vi "getThermocouplesamples.vi"(8 "error in":errorcluster, 11 "params":refnum<class "JSON Value.lvclass">) -> (0 "error out":errorcluster, 3 "data":refnum<class "JSON Value.lvclass">)   [LabVIEW 2017]
uses:
  <vilib>/NI/JSON Support for LabVIEW/JSON Value/JSON Value.lvclass
  <vilib>/DAQmx/read.llb/DAQmx Read (Analog 1D DBL 1Chan NSamp).vi
  <vilib>/NI/JSON Support for LabVIEW/JSON Value/Object/Get Value/Get Value (String).vi
  <vilib>/NI/JSON Support for LabVIEW/JSON Value/Object/Get Value/Get Value (Numeric).vi
  <vilib>/DAQmx/create/channels.llb/DAQmx Create Channel (AI-Temperature-Thermocouple).vi
  <vilib>/DAQmx/configure/timing.llb/DAQmx Timing (Sample Clock).vi
  <vilib>/DAQmx/miscellaneous.llb/DAQmx Fill In Error Info.vi
  <vilib>/NI/JSON Support for LabVIEW/JSON Value/New JSON Value/New JSON (Numeric[]).vi
  <vilib>/NI/JSON Support for LabVIEW/JSON Value/New JSON Value/New JSON (Numeric).vi
  <vilib>/NI/JSON Support for LabVIEW/JSON Value/New JSON Value/New JSON ({Value[]}).vi
  <vilib>/NI/NI JSONRPC Server Framework/Classes/Server/JSONRPC Server.lvclass
  <resource>/objmgr/daqmx.rc
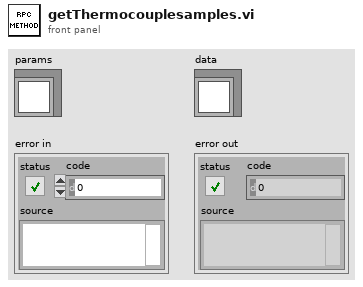
[diagram p1: front panel]
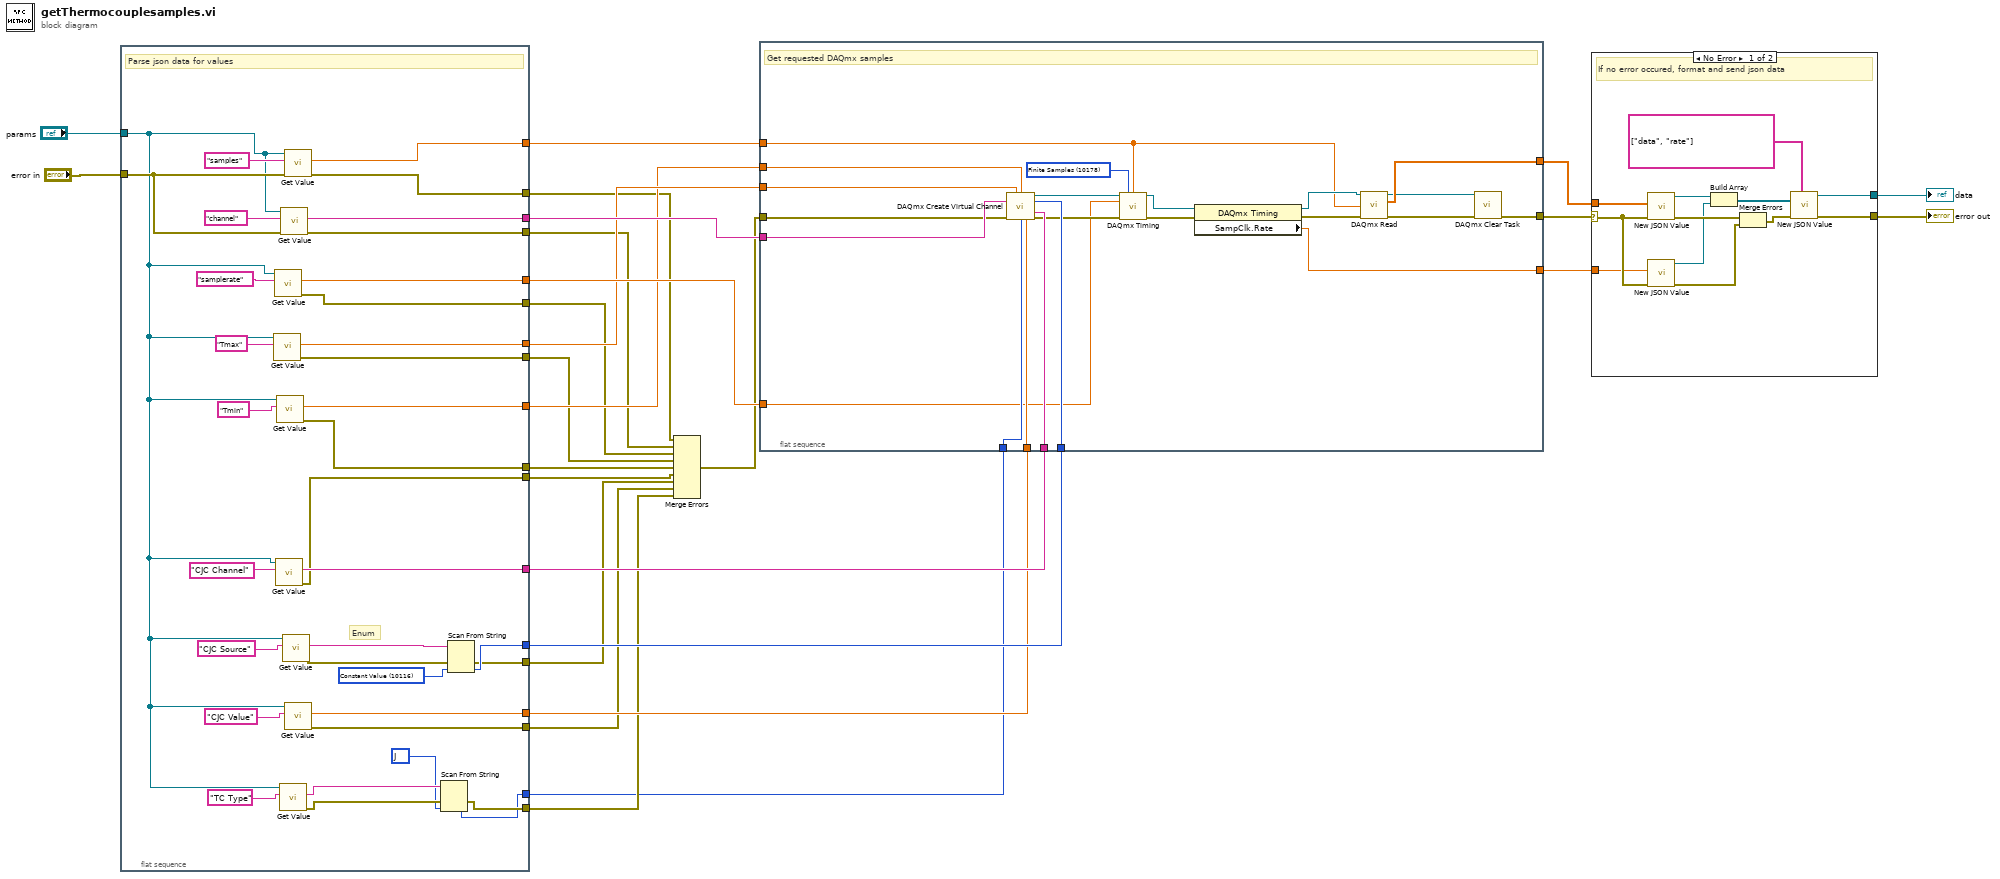
[diagram p0: block diagram]
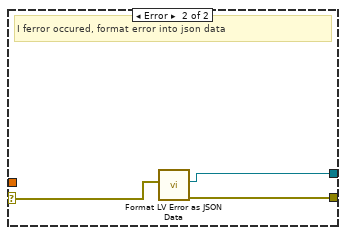
[diagram p2: hidden frame]
diagram:
  n1 = flat-sequence {
    tunnel: "params" -> [w44]
    tunnel: "error in" -> [w57]
    tunnel: [w59] -> w19
    tunnel: [w58] -> w20
    tunnel: [w55] -> w17
    tunnel: [w52] -> w16
    tunnel: [w51] -> w15
    tunnel: [w49] -> w14
    tunnel: [w41] -> w13
    tunnel: [w46] -> w12
    tunnel: [w39] -> w11
    tunnel: [w38] -> w10
    tunnel: [w37] -> w9
    tunnel: [w36] -> w7
    tunnel: [w35] -> w6
    tunnel: [w34] -> w5
    tunnel: [w33] -> w4
    tunnel: [w32] -> w3
    tunnel: [w29] -> w2
    tunnel: [w27] -> w1
    frame #0 {
      w28 = 10072 items=["J"=10072, "K"=10073, "N"=10077, "R"=10082, "S"=10085, "T"=10086, "B"=10047, "E"=10055] ("Thermocouple Type")
      w42 = 10116 items=["Built-In"=10200, "Constant Value"=10116, "Channel"=10113] ("CJC Source")
      # "Enum"
      # "Parse json data for values"
      n2 = call-poly <vilib>:"Get Value.vi"("key"="Tmax", "JSON Value in"=w44) -> ("error out"=w36:errorcluster, "value"=w52:dbl)  [unwired: 8 in]
      n3 = call-poly <vilib>:"Get Value.vi"("key"="samplerate", "JSON Value in"=w44) -> ("error out"=w37:errorcluster, "value"=w55:dbl)  [unwired: 8 in]
      n4 = call-poly <vilib>:"Get Value.vi"("key"="CJC Channel", "JSON Value in"=w44) -> ("error out"=w34:errorcluster, "value"=w49:string)  [unwired: 8 in]
      n5 = call-poly <vilib>:"Get Value.vi"("key"="Tmin", "JSON Value in"=w44) -> ("error out"=w35:errorcluster, "value"=w51:dbl)  [unwired: 8 in]
      n6 = call-poly <vilib>:"Get Value.vi"("key"="TC Type", "JSON Value in"=w44) -> ("error out"=w30:errorcluster, "value"=w31:string)  [unwired: 8 in]
      n7 = call-poly <vilib>:"Get Value.vi"("error in (no error)"=w57, "key"="channel", "JSON Value in"=w44) -> ("error out"=w38:errorcluster, "value"=w58:string)  [unwired: 7 in]
      n8 = call-poly <vilib>:"Get Value.vi"("key"="CJC Source", "JSON Value in"=w44) -> ("error out"=w40:errorcluster, "value"=w43:string)  [unwired: 8 in]
      n9 = call-poly <vilib>:"Get Value.vi"("error in (no error)"=w57, "key"="samples", "JSON Value in"=w44) -> ("error out"=w39:errorcluster, "value"=w59:dbl)  [unwired: 7 in]
      n10 = call-poly <vilib>:"Get Value.vi"("key"="CJC Value", "JSON Value in"=w44) -> ("error out"=w32:errorcluster, "value"=w46:dbl)  [unwired: 8 in]
      n11 = Scan From String(input string=w31, error in=w30, default 1=w28) -> (error out=w29:errorcluster, output 1=w27:i32)  [unwired: 2 in, 2 out]
      n12 = Scan From String(input string=w43, error in=w40, default 1=w42) -> (error out=w33:errorcluster, output 1=w41:i32)  [unwired: 2 in, 2 out]
    }
  }
  n13 = Merge Errors(w11, w10, w9, w7, w6, w5, w4, w3, w2) -> (w8:errorcluster)
  n14 = flat-sequence {
    tunnel: w8 -> [w69]
    tunnel: [w81] -> w22
    tunnel: [w77] -> w21
    tunnel: w20 -> [w72]
    tunnel: w19 -> [w78]
    tunnel: [w74] -> w18
    tunnel: w17 -> [w62]
    tunnel: w16 -> [w71]
    tunnel: w15 -> [w70]
    tunnel: w14 -> [w68]
    tunnel: w13 -> [w67]
    tunnel: w12 -> [w66]
    tunnel: w1 -> [w63]
    frame #0 {
      w65 = 10178 items=["Finite Samples"=10178, "Continuous Samples"=10123, "Hardware Timed Single Point"=12522] ("sample mode")
      # "Get requested DAQmx samples"
      n15 = call-poly <vilib>:"DAQmx Create Virtual Channel.vi"("maximum value"=w71, "minimum value"=w70, "physical channels"=w72, "cjc source"=w67, "cjc channel"=w68, "error in"=w69, "thermocouple type"=w63, "cjc value"=w66) -> ("task out"=w73:refnum<k21>, "error out"=w64:errorcluster)  [unwired: 6 in]
      n16 = call-poly <vilib>:"DAQmx Timing.vi"("task/channels in"=w73, "sample mode"=w65, "samples per channel"=w78, "rate"=w62, "error in"=w64) -> ("task out"=w82:refnum<k21>, "error out"=w83:errorcluster)  [unwired: 9 in]
      n17 = property class="DAQmx Timing"(reference=w82, error in=w83) -> (reference out=w79:refnum<k21>, error out=w80:errorcluster, "SampClk.Rate"=w81:dbl)
      n18 = call-poly <vilib>:"DAQmx Read.vi"("task/channels in"=w79, "number of samples per channel"=w78, "error in"=w80) -> ("task out"=w75:refnum<k21>, "data"=w77:dbl[], "error out"=w76:errorcluster)  [unwired: 10 in]
      n19 = call <vilib>:"DAQmx Clear Task.vi"("task in"=w75, "error in"=w76) -> ("error out"=w74:errorcluster)  [unwired: 13 in]
    }
  }
  n20 = case shown="No Error" w18 {
    selector: w18 -> [w89 w98]
    tunnel: [w94 w96] -> w24
    tunnel: [w88 w97] -> w23
    tunnel: w21 -> [w87 _]
    tunnel: w22 -> [w84 _]
    frame No Error {
      # "If no error occured, format and send json data"
      n21 = call-poly <vilib>:"New JSON Value.vi"("error in (no error)"=w89, "Numeric Array"=w87) -> ("error out"=w95:errorcluster, "JSON Value out"=w93:refnum<class "JSON Value.lvclass">)  [unwired: 8 in]
      n22 = call-poly <vilib>:"New JSON Value.vi"("error in (no error)"=w89, "value"=w84) -> ("error out"=w90:errorcluster, "JSON Value out"=w92:refnum<class "JSON Value.lvclass">)  [unwired: 8 in]
      n23 = Build Array(w93, w92) -> (w86:refnum<class "JSON Value.lvclass">[])
      n24 = Merge Errors(w95, w90) -> (w91:errorcluster)
      n25 = call-poly <vilib>:"New JSON Value.vi"("keys"=string[] ["data", "rate"], "error in (no error)"=w91, "values"=w86) -> ("error out"=w94:errorcluster, "JSON Value out"=w88:refnum<class "JSON Value.lvclass">)  [unwired: 7 in]
    }
    frame Error {
      # "I ferror occured, format error into json data"
      n26 = call <vilib>:"Format LV Error as JSON Data.vi"("error in"=w98) -> ("error out"=w96:errorcluster, "Error Value out"=w97:refnum<class "JSON Value.lvclass">)  [unwired: 9 in]
    }
  }
  "data" <- w23
  "error out" <- w24
